vi "Calculate Position from Angle.vi"(5 "Angle Array":dbl[](array[numeric])=[5.0, 7.0, 10.0, 12.0, 15.0, 17.0, 20.0, 22.0, 25.0, 27.0, 30.0, 37.0, 40.0], 7 "Position Array":i32[](array[numeric])=[100, 142, 184, 226, 268, 290, 332, 374, 416, 458, 500, 542, 584], 11 "Angle":dbl) -> (3 "Sensor Unit Position Out":i32)   [LabVIEW 2020, in "Angler_ACT.lvlib"]
uses:
  Angler_ACT.lvlib
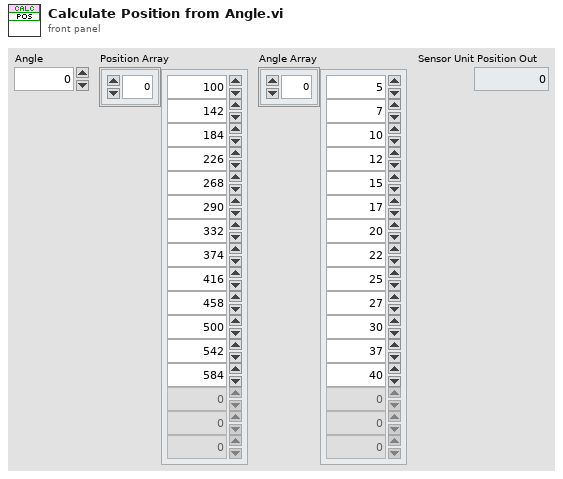
[diagram p1: front panel]
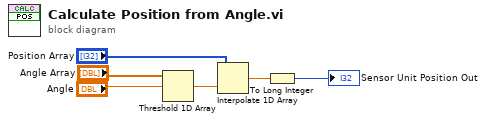
[diagram p0: block diagram]
diagram:
  n1 = Threshold 1D Array(2:"Angle", 3:"Angle Array") -> (0:w6:dbl)  [unwired: 1 in]
  n2 = Interpolate 1D Array(1:w6, 2:"Position Array") -> (0:w2:dbl)
  n3 = To Long Integer(number=w2) -> (32bit integer=→"Sensor Unit Position Out":i32)
